vi "Testing FGV_p.vi"(7 "Set":bool, 8 "error in (no error)":errorcluster, 11 "Value":bool) -> (0 "error out":errorcluster, 3 "Testing?":bool)   [LabVIEW 2016]
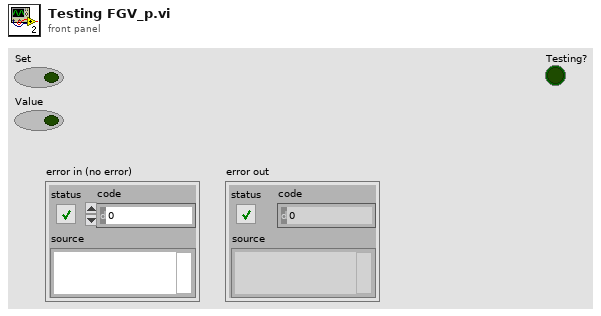
[diagram p1: front panel]
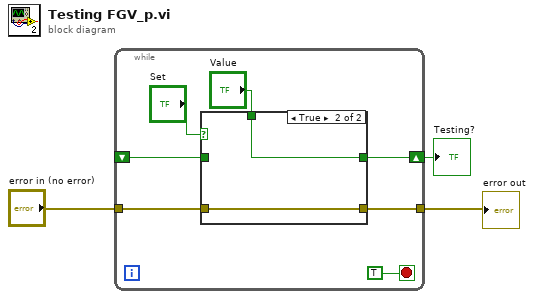
[diagram p0: block diagram]
diagram:
  n1 = while {
    shift-right: [w7] -> w3
    shift-left: _ -> [w6]
    tunnel: "error in (no error)" -> [w5]
    tunnel: [w4] -> w1
    stop <- TRUE stop-if-true
    n2 = case shown="True" "Set" {
      tunnel: "Value" -> [_ w14]
      tunnel: [w12 w14] -> w7
      tunnel: w6 -> [w12 _]
      tunnel: w5 -> [w11 w13]
      tunnel: [w11 w13] -> w4
      frame False {
      }
      frame True {
      }
    }
  }
  "Testing?" <- w3
  "error out" <- w1
